vi "Data Trim Module.vi"(7 "#pixels to save":i32=300, 8 "error in":errorcluster, 9 "start pixel":i32, 10 "#A-lines":i32=2048, 11 "1D Array in":sgl[](array[numeric])) -> (0 "error out":errorcluster, 2 "array for saving":sgl[](array[numeric]))   [LabVIEW 2018]
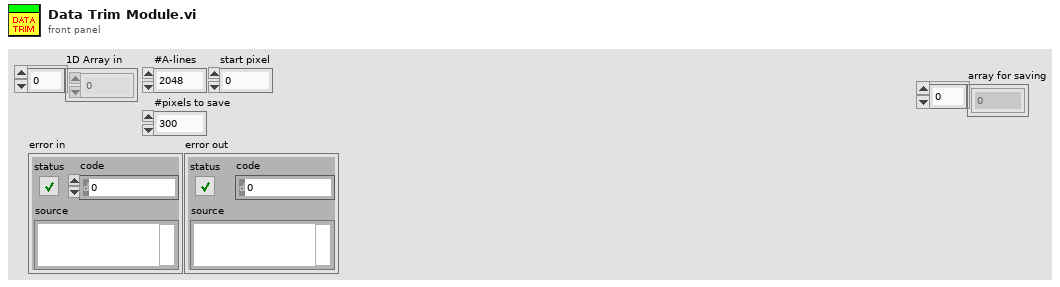
[diagram p1: front panel]
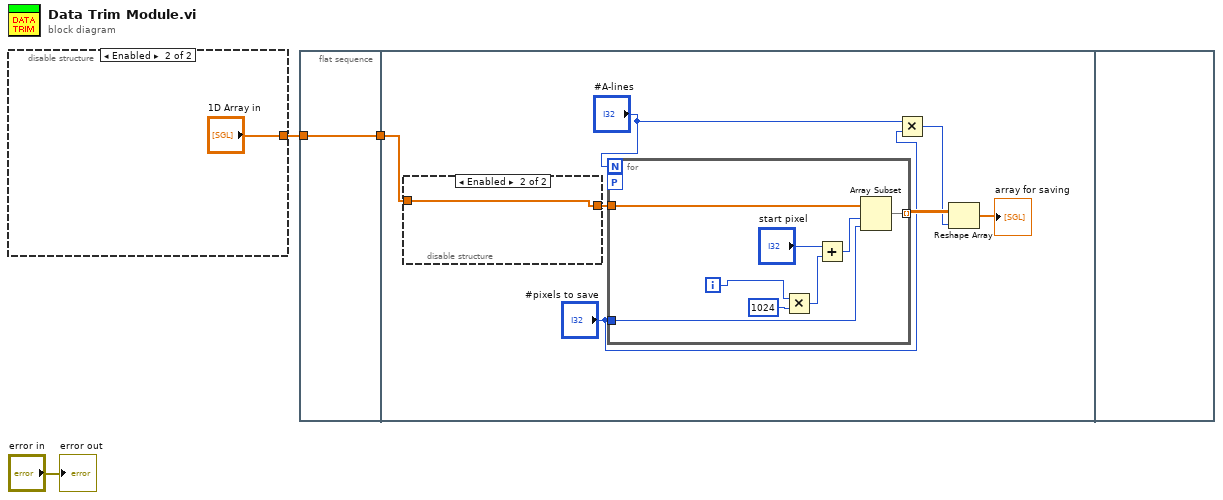
[diagram p0: block diagram]
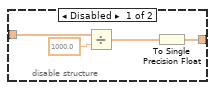
[diagram p2: hidden frame]
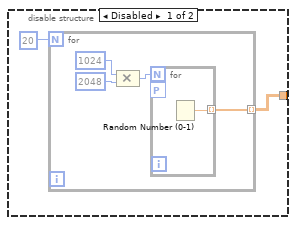
[diagram p3: hidden frame]
diagram:
  n1 = disable-structure shown="Enabled" {
    disable-tunnel: [w4 "1D Array in"] -> w1
    frame Disabled {
      n2 = for {
        N: 20 -> [_]
        tunnel: [w6] -> w4 mode=indexing
        n3 = Compound Arithmetic op=MULTIPLY(1024, 2048) -> (w7:i32)
        n4 = for {
          N: w7 -> [_]
          tunnel: [w10] -> w6 mode=indexing
          workers-P: _ -> [_]
          n5 = Random Number (0-1)() -> (number: 0 to 1=w10:dbl)
        }
      }
    }
    frame Enabled {
    }
  }
  n6 = flat-sequence {
    tunnel: w1 -> [w12]
    tunnel: [w12] -> w3
    tunnel: w3 -> [w19]
    frame #0 {
    }
    frame #1 {
      n7 = disable-structure shown="Enabled" {
        disable-tunnel: w19 -> [w31 w32]
        disable-tunnel: [w28 w32] -> w18
        frame Disabled {
          n8 = Divide(x=w31, y=sgl 1000.0) -> (x/y=w29:sgl[])
          n9 = To Single Precision Float(number=w29) -> (single precision float=w28:sgl[])
        }
        frame Enabled {
        }
      }
      n10 = for {
        N: "#A-lines" -> [_]
        tunnel: w18 -> [w26]
        workers-P: _ -> [_]
        tunnel: [w25] -> w17 mode=indexing
        tunnel: "#pixels to save" -> [w24]
        i -> [w20]
        n11 = Multiply(x=w20, y=1024) -> (x*y=w22:i32)
        n12 = Add(x="start pixel", y=w22) -> (x+y=w21:i32)
        n13 = Array Subset(array=w26, index=w21, length=w24) -> (w25:sgl[])
      }
      n14 = Multiply(x="#A-lines", y="#pixels to save") -> (x*y=w14:i32)
      n15 = Reshape Array(w17, w14) -> (→"array for saving":sgl[])
    }
    frame #2 {
    }
  }
  "error out" <- "error in"
